vi "Exercise 2.3 - Decision Making and Saving Data.vi"() -> ()   [LabVIEW 2024]
panel:
  in  "Limit":dbl(knob) scale=0.0..500.0
  out "Frequency":dbl
  out "Amplitude":dbl
  in  "stop":bool
  out "Filtered Signal":dynamicdata(graph)
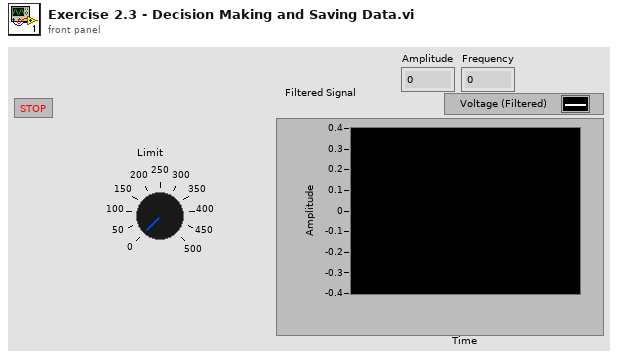
[diagram p1: front panel]
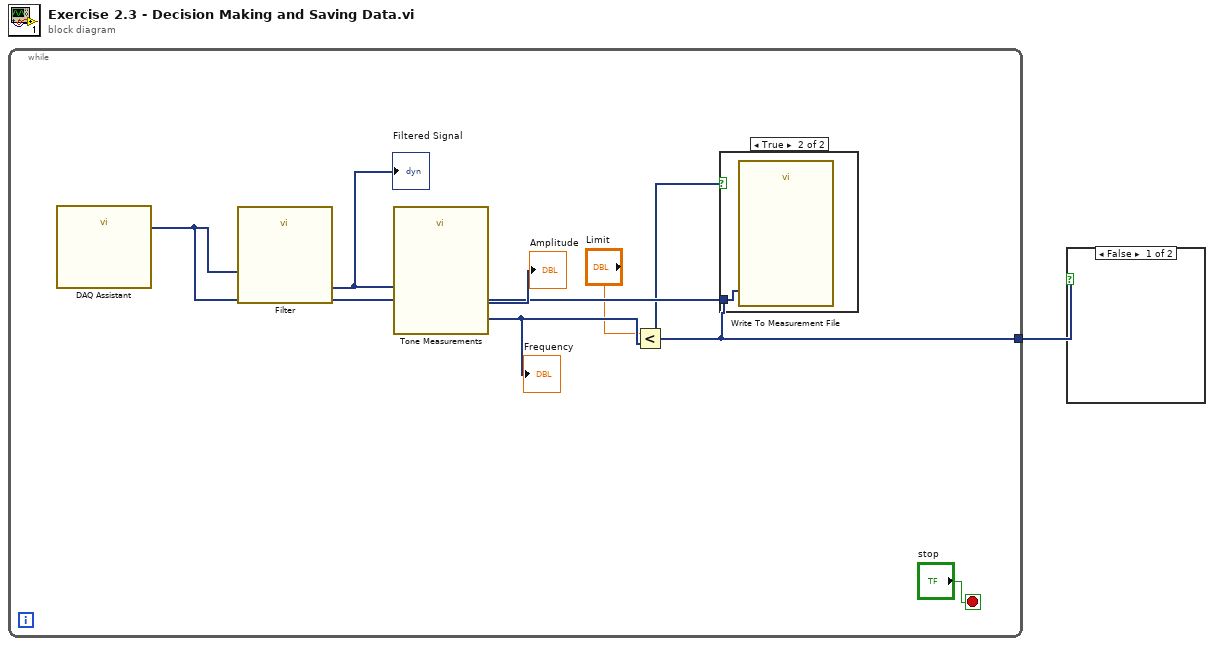
[diagram p0: block diagram]
diagram:
  n1 = while {
    tunnel: [w2] -> w1
    stop <- "stop" stop-if-true
    n2 = call "DAQ Assistant"() -> ("data"=w5:dynamicdata)  [unwired: 16 in, 3 out]
    n3 = call "Filter"("Signal"=w5) -> ("Filtered Signal"=w6:dynamicdata)  [unwired: 9 in, 1 out]
    "Filtered Signal" <- w6
    n4 = call "Tone Measurements"("Signals"=w6) -> ("Frequency"=w4:dynamicdata, "Amplitude"=→"Amplitude":dynamicdata)  [unwired: 8 in, 1 out]
    "Frequency" <- w4
    n5 = Less?(x="Limit", y=w4) -> (x < y?=w2:dynamicdata)
    n6 = case shown="True" w2 {
      tunnel: w5 -> [_ w9]
      tunnel: w2 -> [_ _]
      frame False {
      }
      frame True {
        n7 = call "Write To Measurement File"("Signals"=w9) -> ()  [unwired: 16 in, 3 out]
      }
    }
  }
  n8 = case shown="False" w1 {
    frame False {
    }
    frame True {
    }
  }
